vi "CircularRadius.vi"(0 "controller in":refnum<k24>, 1 "axis 1 name":string, 2 "axis 1 endpoint":dbl, 3 "axis 2 name":string, 4 "axis 2 endpoint":dbl, 5 "error in (no error)":errorcluster, 6 "speed":dbl, 7 "radius":dbl, 8 "direction":u16(ring) items=["Clockwise", "Counter-clockwise"], 9 "taskId":i32(ring) items=["TLibrary", "T01", "T02", "T03", "T04", "T05", "T06", "T07", "T08", "T09", "T10", "T11", "T12", "T13", "T14", "T15", "T16", "T17", "T18", "T19", "T20", "T21", "T22", "T23", "T24", "T25", "T26", "T27", "T28", "T29", "T30", "T31"], 11 "return immediately":bool) -> (14 "controller out":refnum<k24>, 19 "error out":errorcluster)   [LabVIEW 2016]
uses:
  C:/Users/TTUHEP/Documents/LabVIEW/2010/Bin/Aerotech.A3200.dll
  Bin/Aerotech.A3200.dll
  C:/Users/TTUHEP/Documents/LabVIEW/2010/Bin/Aerotech.A3200.LabVIEW.dll
  Bin/Aerotech.A3200.LabVIEW.dll
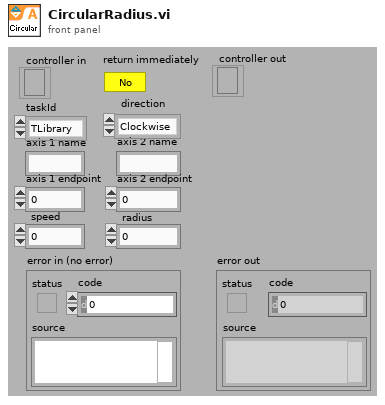
[diagram p1: front panel]
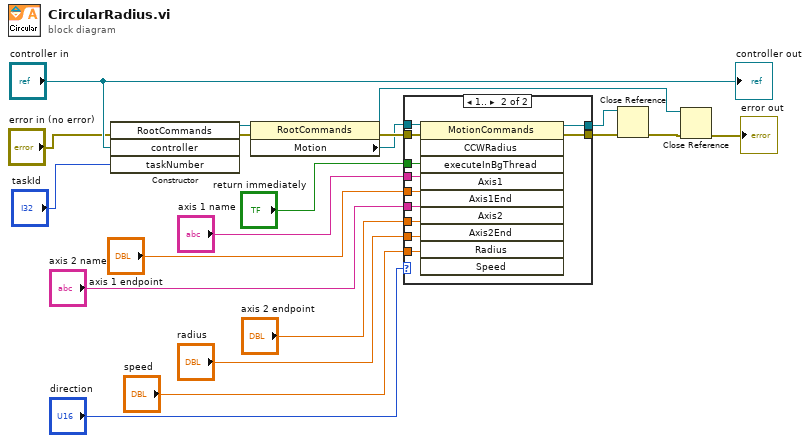
[diagram p0: block diagram]
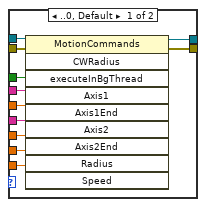
[diagram p2: hidden frame]
diagram:
  n1 = constructor class="RootCommands"(error in="error in (no error)", "controller"="controller in", "taskNumber"="taskId") -> (reference out=w4:refnum<k24>, error out=w5:errorcluster)  [unwired: 2 in, 3 out]
  n2 = property class="RootCommands"(reference=w4, error in=w5) -> (reference out=w9:refnum<k24>, error out=w3:errorcluster, "Motion"=w2:refnum<k24>)
  n3 = case shown="1.." "direction" {
    tunnel: [w31 w40] -> w7
    tunnel: [w30 w39] -> w6
    tunnel: w3 -> [w29 w42]
    tunnel: w2 -> [w28 w41]
    tunnel: "speed" -> [w27 w38]
    tunnel: "radius" -> [w26 w37]
    tunnel: "axis 2 endpoint" -> [w25 w36]
    tunnel: "axis 1 name" -> [w24 w33]
    tunnel: "axis 1 endpoint" -> [w23 w34]
    tunnel: "axis 2 name" -> [w22 w35]
    tunnel: "return immediately" -> [w21 w32]
    frame ..0, Default {
      n4 = invoke class="MotionCommands" method="CWRadius"(reference=w28, error in=w29, "executeInBgThread"=w21, "Axis1"=w24, "Axis1End"=w23, "Axis2"=w22, "Axis2End"=w25, "Radius"=w26, "Speed"=w27) -> (reference out=w31:refnum<k24>, error out=w30:errorcluster)  [unwired: 1 in, 8 out]
    }
    frame 1.. {
      n5 = invoke class="MotionCommands" method="CCWRadius"(reference=w41, error in=w42, "executeInBgThread"=w32, "Axis1"=w33, "Axis1End"=w34, "Axis2"=w35, "Axis2End"=w36, "Radius"=w37, "Speed"=w38) -> (reference out=w40:refnum<k24>, error out=w39:errorcluster)  [unwired: 1 in, 8 out]
    }
  }
  n6 = Close Reference(reference=w7, error in (no error)=w6) -> (error out=w8:errorcluster)
  n7 = Close Reference(reference=w9, error in (no error)=w8) -> (error out=→"error out":errorcluster)
  "controller out" <- "controller in"
